vi "_RT_Pub_EC_Str2I32Arr.vi"(1 "input string":string) -> (0 "appended array":i32[](array[numeric]))   [LabVIEW 2018]
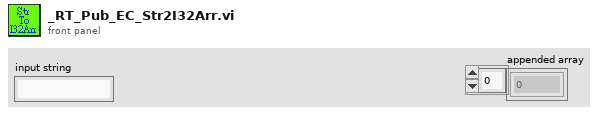
[diagram p1: front panel]
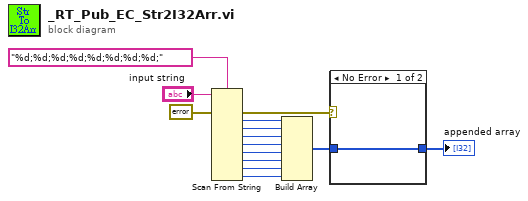
[diagram p0: block diagram]
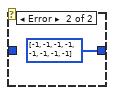
[diagram p2: hidden frame]
diagram:
  n1 = Scan From String(format string="%d;%d;%d;%d;%d;%d;%d;%d;", input string="input string", error in=errorcluster {"status"=FALSE, "code"=0, "source"=""}) -> (error out=w3:errorcluster, output 1=w13:i32, output 2=w12:i32, output 3=w11:i32, output 4=w10:i32, output 5=w9:i32, output 6=w8:i32, output 7=w7:i32, output 8=w6:i32)  [unwired: 9 in, 2 out]
  n2 = Build Array(w13, w12, w11, w10, w9, w8, w7, w6) -> (w2:i32[])
  n3 = case shown="No Error" w3 {
    tunnel: w2 -> [w15 _]
    tunnel: [w15 i32[] [-1, -1, -1, -1, -1, -1, -1, -1]] -> w1
    frame No Error {
    }
    frame Error {
    }
  }
  "appended array" <- w1
